vi "response.free.vi"(8 "error in (no error)":errorcluster, 11 "handle":cluster{}) -> (0 "error out":errorcluster, 3 "function return":i32)   [LabVIEW 2020, in "reqwest-labview.lvlib"]
doc: "Discards a stored response without reading it; call this in error-handling paths where a request succeeded but the response body is not needed.\n\n\n\n\n\n\nint http_free_response(unsigned long long handle);"
uses:
  reqwest-labview.lvlib
  http_rs_labview.dll
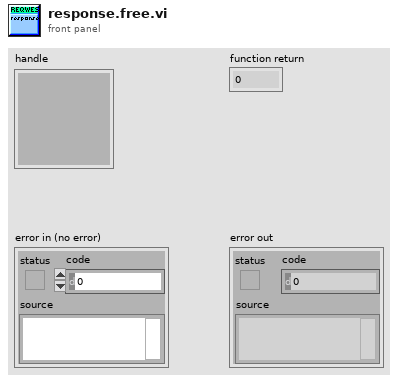
[diagram p1: front panel]
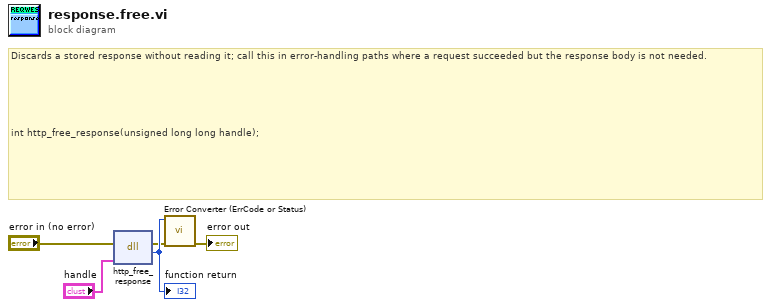
[diagram p0: block diagram]
diagram:
  # "Discards a stored response without reading it; call this in error-handling paths where a request succeeded but the response body is not needed.\n\n\n\n\n\n\nint http_free_response(unsigned long long handle);"
  n1 = dll-call lib="C:/code/reqwest-labview/lv-src/shared-library/http_rs_labview.*" fn="http_free_response"(error in="error in (no error)", "handle"="handle") -> (error out=w2:errorcluster, w5:i32)  [unwired: 3 in, 1 out]
  "function return" <- w5
  n2 = call "Error Converter (ErrCode or Status).vi"("error in (no error)"=w2, "error code"=w5) -> ("error out"=→"error out":errorcluster)  [unwired: 9 in]
